vi "Write Weight.vi"(8 "error in (no error)":errorcluster, 10 "Weight":cdb[][](array[numeric]), 11 "ConfigProc in":refnum<class "ConfigProc.lvclass">) -> (0 "error out":errorcluster, 3 "ConfigProc out":refnum<class "ConfigProc.lvclass">)   [LabVIEW 2017, in "ConfigProc.lvclass"]
uses:
  ConfigProc.lvclass
  ConfigProc.lvclass/ConfigProc.ctl
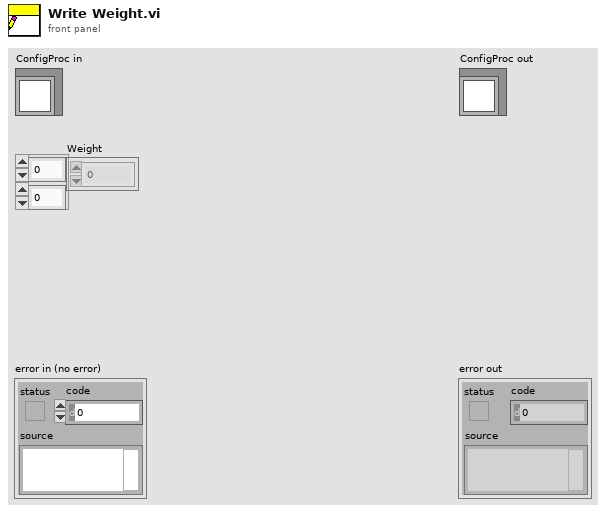
[diagram p1: front panel]
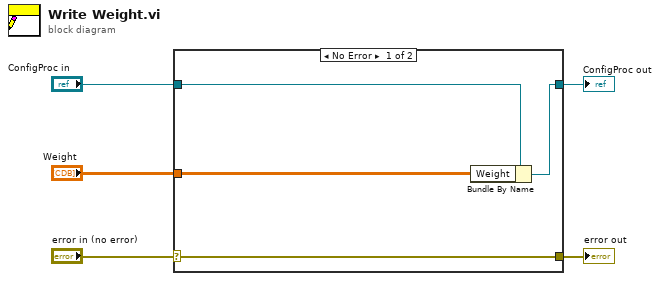
[diagram p0: block diagram]
diagram:
  n1 = case shown="No Error" "error in (no error)" {
    selector: "error in (no error)" -> [w9 w10]
    tunnel: [w9 w10] -> w4
    tunnel: [w7 w11] -> w2
    tunnel: "ConfigProc in" -> [w8 w11]
    tunnel: "Weight" -> [w6 _]
    frame No Error {
      n2 = Bundle By Name(cluster=w8, "Weight"=w6) -> (w7:refnum<class "ConfigProc.lvclass">)
    }
    frame Error {
    }
  }
  "error out" <- w4
  "ConfigProc out" <- w2
